vi "ModelParameterValueGet.vi"(9 "Target":string, 10 "Parameter":string) -> (0 "error out":errorcluster, 1 "Target out":string, 2 "Parameter name out":string, 3 "Value":dbl)   [LabVIEW 2015, in "ni-veristand-steps-runtime-lib.lvlib"]
uses:
  ni-veristand-steps-runtime-lib.lvlib
  <vilib>/NI Veristand/Execution/ModelManager/NI VeriStand - Get Single Parameter Value.vi
  <vilib>/NI Veristand/Execution/ModelManager/NI_VS ModelManager ExecutionAPI.lvlib
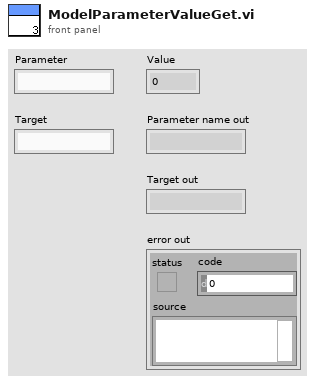
[diagram p1: front panel]
types:
  T1 = typedef "ni-veristand-steps-runtime-lib.lvlib/VeriStand dotNet References.ctl" = cluster{"Project Ref":refnum<k24>, "ModelManager":T2, "AlarmManager":T3, "ChannelFault":T4, "WorkspaceManager":T5}
  T2 = typedef "NI_VS ModelManager ExecutionAPI.lvlib/ModelManagerAPI.ctl" = refnum<k24>
  T3 = typedef "NI_VS AlarmManager ExecutionAPI.lvlib/AlarmManagerAPI.ctl" = refnum<k24>
  T4 = typedef "NI_VS ChannelFault ExecutionAPI.lvlib/ChannelFaultAPI.ctl" = refnum<k24>
  T5 = typedef "NI_VS Workspace ExecutionAPI.lvlib/WorkspaceAPI.ctl" = refnum<k24>
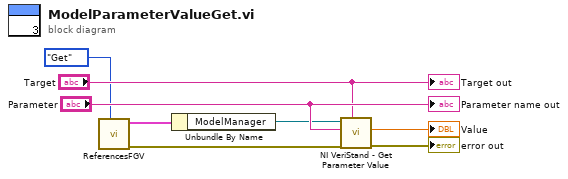
[diagram p0: block diagram]
diagram:
  n1 = call "ReferencesFGV.vi"("Get/Set"=enum16{"Get", "Set"}."Get") -> ("error out"=w3:errorcluster, "VeriStand dotNET Refs out"=w2:T1)  [unwired: 9 in]
  n2 = Unbundle By Name(w2) -> ("ModelManager"=w1:T2)
  n3 = call-poly <vilib>:"NI VeriStand - Get Parameter Value.vi"("Target"="Target", "error in (no error)"=w3, "Parameter"="Parameter", "ModelManager in"=w1) -> ("error out"=→"error out":errorcluster, "Value"=→"Value":dbl)  [unwired: 5 in, 1 out]
  "Parameter name out" <- "Parameter"
  "Target out" <- "Target"
